vi "Get All Indicator Labels.vi"(8 "error in":errorcluster, 11 "Class in":refnum<class>) -> (0 "error out":errorcluster, 2 "Labels":string[](array[string]), 3 "Class out":refnum<class>)   [LabVIEW 2023, in "Label-Driven UI.lvlib"]
doc: "VI가 가진 모든 인디케이터의 라벨들을 얻습니다."
uses:
  Label-Driven UI.lvlib
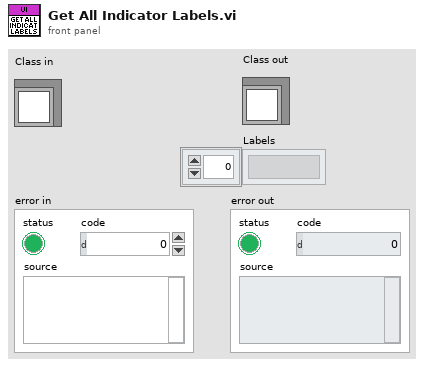
[diagram p1: front panel]
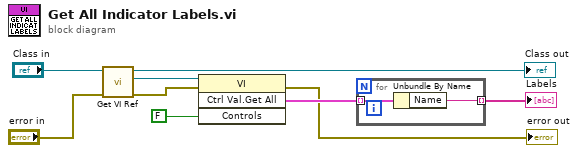
[diagram p0: block diagram]
diagram:
  n1 = call "Get VI Ref.vi"("error in"="error in", "Class in"="Class in") -> ("error out"=w7:errorcluster, "VI Refnum"=w9:refnum<vi>, "Class out"=→"Class out":refnum<class>)  [unwired: 7 in]
  n2 = invoke class="VI" method="Ctrl Val.Get All"(reference=w9, error in=w7, "Controls"=FALSE) -> (error out=→"error out":errorcluster, "Get All Control Values Variant"=w4:cluster{"Name":string, "Variant Data":variant}[])  [unwired: 1 in, 2 out]
  n3 = for {
    tunnel: w4 -> [w11] mode=indexing
    tunnel: [w10] -> w3 mode=indexing
    n4 = Unbundle By Name(w11) -> ("Name"=w10:string)
  }
  "Labels" <- w3
